vi "SavePictureData.vi"(6 "File Path":path, 8 "error in (no error)":errorcluster, 9 "Exposure":dbl, 10 "Index":u32, 11 "Name":string) -> (0 "error out":errorcluster)   [LabVIEW 2013]
panel:
  out "appended path":path
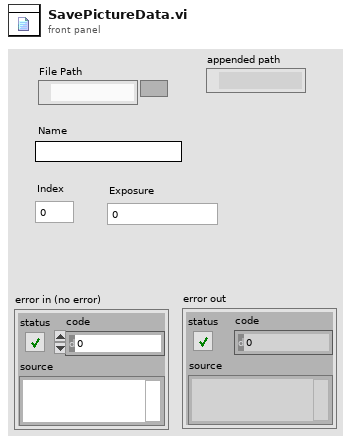
[diagram p1: front panel]
types:
  T1 = enum16{"open", "replace", "create", "open or create", "replace or create", "replace or create with confirmation"}
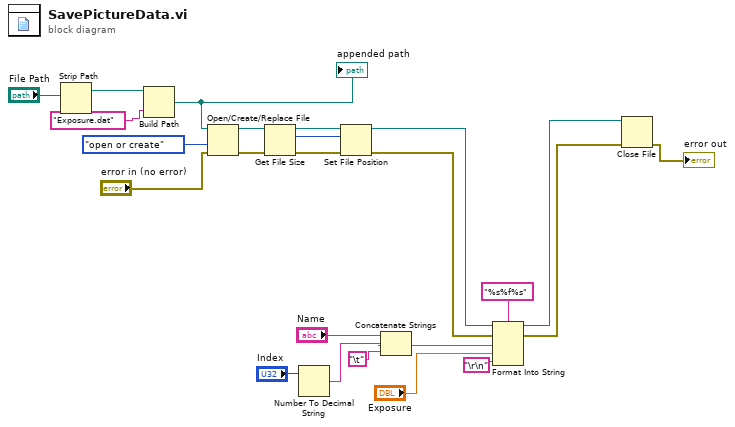
[diagram p0: block diagram]
diagram:
  n1 = Strip Path(path="File Path") -> (stripped path=w3:path)  [unwired: 1 out]
  n2 = Build Path(base path=w3, name or relative path="Exposure.dat") -> (appended path=w4:path)
  "appended path" <- w4
  n3 = Open/Create/Replace File(file path (use dialog)=w4, error in="error in (no error)", operation (0:open)=T1."open or create") -> (refnum out=w16:refnum<file>, error out=w11:errorcluster)  [unwired: 3 in, 1 out]
  n4 = Get File Size(file=w16, error in=w11) -> (refnum out=w15:refnum<file>, size (in bytes)=w14:i64, 0:w10:errorcluster)
  n5 = Number To Decimal String(number="Index") -> (decimal integer string=w21:string)  [unwired: 1 in]
  n6 = Set File Position(offset (in bytes) (0)=w14, refnum=w15, error in=w10) -> (refnum out=w17:refnum<file>, error out=w7:errorcluster)  [unwired: 1 in]
  n7 = Concatenate Strings("Name", w21, "\t") -> (w20:string)
  n8 = Format Into String(format string="%s%f%s" ("format (%.3f)"), initial string=w17, error in=w7, w20, "Exposure", "\r\n") -> (resulting string=w23:refnum<file>, error out=w22:errorcluster)
  n9 = Close File(refnum=w23, error in=w22) -> (error out=→"error out":errorcluster)  [unwired: 1 out]
